vi "Process RS232 Messages.vi"(8 "error in (no error)":errorcluster, 10 "rt fifo":refnum<k33>, 11 "BMS RS232 STRING":string) -> (0 "error out":errorcluster, 2 "rt fifo out":refnum<k33>)   [LabVIEW 2015]
uses:
  1dstr.ctl
  <vilib>/RioEmbeddedCAN/RioEmbeddedCAN.llb/CANFrameControl.ctl
  Global Data.vi
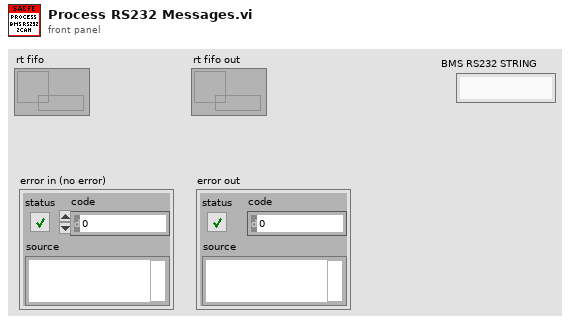
[diagram p1: front panel]
types:
  T1 = typedef "1dstr.ctl" = string[]
  T2 = typedef "CANFrameControl.ctl" = cluster{"identifier":u32, "extended?":bool, "type":u8, "payload":u8[]}
  T3 = typedef "BMS Telemetry.ctl" = cluster{"bBMSIgnition":bool, "bBMSChargerMains":bool, "bBMSFastCharge":bool, "bBMSChargerEnabled":bool, "eBMSCarState":enum16{"Off", "On, Not Charging", "Charging", "Charging Finished", "Charging Error"}, "eBMSChargingState":enum16{"Disconnected", "Pre-charging", "Main Charging", "Balancing", "Charging Finished OK", "Charging Error"}, "tBMSChargeStage":u16, "eBMSLastChargeError":enum16{"No Error", "No Cell Communication", "No Cell Communication - Non CAN Charger", "Maximum charging stage duration expired", "Cell Communication Lost during Charge", "Cannot set balancing voltage", "Cell temps too high", "No Comms so can't determine temp", "# of Cells Mismatch", "Cells Overvoltage", "Cell Protection Event occured."}, "NBMSNumCells":u8, "bBMSUnderVProtection":bool, "bBMSOverVProtection":bool, "bBMSOverTProtection":bool, "bBMSLeakageProtection":bool, "bBMSNoCellCommsError":bool, "bBMSLowVReduction":bool, "bBMSHighTReduction":bool, "VCellMin":dbl, "VCellMax":dbl, "VCellMean":dbl, "VTotal":dbl, "TCellMin":dbl, "TCellMax":dbl, "TCellMean":dbl, "VCells":cluster{"[51]":dbl, "[53]":dbl, "[54]":dbl, "[55]":dbl, "[56]":dbl, "[57]":dbl, "[58]":dbl, "[59]":dbl, "[60]":dbl, "[61]":dbl, "[62]":dbl, "[63]":dbl, "[64]":dbl, "[65]":dbl, "[66]":dbl, "[67]":dbl, "[34]":dbl, "[35]":dbl, "[36]":dbl, "[37]":dbl, "[38]":dbl, "[39]":dbl, "[40]":dbl, "[41]":dbl, "[42]":dbl, "[43]":dbl, "[44]":dbl, "[45]":dbl, "[46]":dbl, "[47]":dbl, "[48]":dbl, "[49]":dbl, "[50]":dbl, "[17]":dbl, "[18]":dbl, "[19]":dbl, "[20]":dbl, "[21]":dbl, "[22]":dbl, "[23]":dbl, "[24]":dbl, "[25]":dbl, "[26]":dbl, "[27]":dbl, "[28]":dbl, "[29]":dbl, "[30]":dbl, "[31]":dbl, "[32]":dbl, "[33]":dbl, "[0]":dbl, "[1]":dbl, "[2]":dbl, "[3]":dbl, "[4]":dbl, "[5]":dbl, "[6]":dbl, "[7]":dbl, "[8]":dbl, "[9]":dbl, "[10]":dbl, "[11]":dbl, "[12]":dbl, "[13]":dbl, "[14]":dbl, "[15]":dbl, "[16]":dbl, "[52] 2":dbl}, "TBMSCells":cluster{"[55]":dbl, "[56]":dbl, "[57]":dbl, "[58]":dbl, "[59]":dbl, "[60]":dbl, "[61]":dbl, "[62]":dbl, "[63]":dbl, "[64]":dbl, "[65]":dbl, "[66]":dbl, "[67]":dbl, "[68]":dbl, "[69]":dbl, "[70]":dbl, "[17]":dbl, "[38]":dbl, "[39]":dbl, "[40]":dbl, "[41]":dbl, "[42]":dbl, "[43]":dbl, "[44]":dbl, "[45]":dbl, "[46]":dbl, "[47]":dbl, "[48]":dbl, "[49]":dbl, "[50]":dbl, "[51]":dbl, "[52]":dbl, "[53]":dbl, "[54]":dbl, "[21]":dbl, "[22]":dbl, "[23]":dbl, "[24]":dbl, "[25]":dbl, "[26]":dbl, "[27]":dbl, "[28]":dbl, "[29]":dbl, "[30]":dbl, "[31]":dbl, "[32]":dbl, "[33]":dbl, "[34]":dbl, "[35]":dbl, "[36]":dbl, "[37]":dbl, "[0]":dbl, "[1]":dbl, "[2]":dbl, "[3]":dbl, "[4]":dbl, "[5]":dbl, "[6]":dbl, "[7]":dbl, "[8]":dbl, "[9]":dbl, "[10]":dbl, "[11]":dbl, "[12]":dbl, "[13]":dbl, "[14]":dbl, "[15]":dbl, "[16]":dbl}, "bChargerConnected":bool, "VChargerSetpoint":dbl, "IChargerSetpoint":dbl, "VChargerActual":dbl, "IChargerActual":dbl, "BCells":cluster{"[51]":dbl, "[52]":dbl, "[53]":dbl, "[54]":dbl, "[55]":dbl, "[56]":dbl, "[57]":dbl, "[58]":dbl, "[59]":dbl, "[60]":dbl, "[61]":dbl, "[62]":dbl, "[63]":dbl, "[64]":dbl, "[65]":dbl, "[66]":dbl, "[67]":dbl, "[34]":dbl, "[35]":dbl, "[36]":dbl, "[37]":dbl, "[38]":dbl, "[39]":dbl, "[40]":dbl, "[41]":dbl, "[42]":dbl, "[43]":dbl, "[44]":dbl, "[45]":dbl, "[46]":dbl, "[47]":dbl, "[48]":dbl, "[49]":dbl, "[50]":dbl, "[17]":dbl, "[18]":dbl, "[19]":dbl, "[20]":dbl, "[21]":dbl, "[22]":dbl, "[23]":dbl, "[24]":dbl, "[25]":dbl, "[26]":dbl, "[27]":dbl, "[28]":dbl, "[29]":dbl, "[30]":dbl, "[31]":dbl, "[32]":dbl, "[33]":dbl, "[0]":dbl, "[1]":dbl, "[2]":dbl, "[3]":dbl, "[4]":dbl, "[5]":dbl, "[6]":dbl, "[7]":dbl, "[8]":dbl, "[9]":dbl, "[10]":dbl, "[11]":dbl, "[12]":dbl, "[13]":dbl, "[14]":dbl, "[15]":dbl, "[16]":dbl}, "bNewVCellMinSample":bool, "Battery Temp":cluster{"[0]":dbl, "[1]":dbl, "[2]":dbl, "[3]":dbl, "[4]":dbl, "[5]":dbl, "[6]":dbl, "[7]":dbl, "[8]":dbl, "[9]":dbl, "[10]":dbl, "[11]":dbl, "[12]":dbl, "[13]":dbl, "[14]":dbl, "[15]":dbl, "[16]":dbl, "[0] 6":dbl, "[17]":dbl, "[18]":dbl, "[19]":dbl, "[20]":dbl, "[21]":dbl, "[22]":dbl, "[23]":dbl, "[24]":dbl, "[25]":dbl, "[26]":dbl, "[27]":dbl, "[28]":dbl, "[29]":dbl, "[30]":dbl, "[31]":dbl, "[32]":dbl, "[33]":dbl, "[17] 6":dbl, "[34]":dbl, "[35]":dbl, "[36]":dbl, "[37]":dbl, "[38]":dbl, "[39]":dbl, "[40]":dbl, "[41]":dbl, "[42]":dbl, "[43]":dbl, "[44]":dbl, "[45]":dbl, "[46]":dbl, "[47]":dbl, "[48]":dbl, "[49]":dbl, "[50]":dbl, "[34] 6":dbl, "[51]":dbl, "[52] 2":dbl, "[53]":dbl, "[54]":dbl, "[55]":dbl, "[56]":dbl, "[57]":dbl, "[58]":dbl, "[59]":dbl, "[60]":dbl, "[61]":dbl, "[62]":dbl, "[63]":dbl, "[64]":dbl, "[65]":dbl, "[66]":dbl, "[67]":dbl, "[51] 6":dbl, "[0] 2":dbl, "[1] 2":dbl, "[2] 2":dbl, "[3] 2":dbl, "[4] 2":dbl, "[5] 2":dbl, "[6] 2":dbl, "[7] 2":dbl, "[8] 2":dbl, "[9] 2":dbl, "[10] 2":dbl, "[11] 2":dbl, "[12] 2":dbl, "[13] 2":dbl, "[14] 2":dbl, "[15] 2":dbl, "[16] 2":dbl, "[0] 7":dbl, "[17] 2":dbl, "[18] 2":dbl, "[19] 2":dbl, "[20] 2":dbl, "[21] 2":dbl, "[22] 2":dbl, "[23] 2":dbl, "[24] 2":dbl, "[25] 2":dbl, "[26] 2":dbl, "[27] 2":dbl, "[28] 2":dbl, "[29] 2":dbl, "[30] 2":dbl, "[31] 2":dbl, "[32] 2":dbl, "[33] 2":dbl, "[17] 7":dbl, "[34] 2":dbl, "[35] 2":dbl, "[36] 2":dbl, "[37] 2":dbl, "[38] 2":dbl, "[39] 2":dbl, "[40] 2":dbl, "[41] 2":dbl, "[42] 2":dbl, "[43] 2":dbl, "[44] 2":dbl, "[45] 2":dbl, "[46] 2":dbl, "[47] 2":dbl, "[48] 2":dbl, "[49] 2":dbl, "[50] 2":dbl, "[34] 7":dbl, "[51] 2":dbl, "[52] 3":dbl, "[53] 2":dbl, "[54] 2":dbl, "[55] 2":dbl, "[56] 2":dbl, "[57] 2":dbl, "[58] 2":dbl, "[59] 2":dbl, "[60] 2":dbl, "[61] 2":dbl, "[62] 2":dbl, "[63] 2":dbl, "[64] 2":dbl, "[65] 2":dbl, "[66] 2":dbl, "[67] 2":dbl, "[51] 7":dbl, "[0] 3":dbl, "[1] 3":dbl, "[2] 3":dbl, "[3] 3":dbl, "[4] 3":dbl, "[5] 3":dbl, "[6] 3":dbl, "[7] 3":dbl, "[8] 3":dbl, "[9] 3":dbl, "[10] 3":dbl, "[11] 3":dbl, "[12] 3":dbl, "[13] 3":dbl, "[14] 3":dbl, "[15] 3":dbl, "[16] 3":dbl, "[0] 8":dbl, "[17] 3":dbl, "[18] 3":dbl, "[19] 3":dbl, "[20] 3":dbl, "[21] 3":dbl, "[22] 3":dbl, "[23] 3":dbl, "[24] 3":dbl, "[25] 3":dbl, "[26] 3":dbl, "[27] 3":dbl, "[28] 3":dbl, "[29] 3":dbl, "[30] 3":dbl, "[31] 3":dbl, "[32] 3":dbl, "[33] 3":dbl, "[17] 8":dbl, "[34] 3":dbl, "[35] 3":dbl, "[36] 3":dbl, "[37] 3":dbl, "[38] 3":dbl, "[39] 3":dbl, "[40] 3":dbl, "[41] 3":dbl, "[42] 3":dbl, "[43] 3":dbl, "[44] 3":dbl, "[45] 3":dbl, "[46] 3":dbl, "[47] 3":dbl, "[48] 3":dbl, "[49] 3":dbl, "[50] 3":dbl, "[34] 8":dbl, "[51] 3":dbl, "[52] 4":dbl, "[53] 3":dbl, "[54] 3":dbl, "[55] 3":dbl, "[56] 3":dbl, "[57] 3":dbl, "[58] 3":dbl, "[59] 3":dbl, "[60] 3":dbl, "[61] 3":dbl, "[62] 3":dbl, "[63] 3":dbl, "[64] 3":dbl, "[65] 3":dbl, "[66] 3":dbl, "[67] 3":dbl, "[51] 8":dbl, "[0] 4":dbl, "[1] 4":dbl, "[2] 4":dbl, "[3] 4":dbl, "[4] 4":dbl, "[5] 4":dbl, "[6] 4":dbl, "[7] 4":dbl, "[8] 4":dbl, "[9] 4":dbl, "[10] 4":dbl, "[11] 4":dbl, "[12] 4":dbl, "[13] 4":dbl, "[14] 4":dbl, "[15] 4":dbl, "[16] 4":dbl, "[0] 9":dbl, "[17] 4":dbl, "[18] 4":dbl, "[19] 4":dbl, "[20] 4":dbl, "[21] 4":dbl, "[22] 4":dbl, "[23] 4":dbl, "[24] 4":dbl, "[25] 4":dbl, "[26] 4":dbl, "[27] 4":dbl, "[28] 4":dbl, "[29] 4":dbl, "[30] 4":dbl, "[31] 4":dbl, "[32] 4":dbl, "[33] 4":dbl, "[17] 9":dbl, "[34] 4":dbl, "[35] 4":dbl, "[36] 4":dbl, "[37] 4":dbl, "[38] 4":dbl, "[39] 4":dbl, "[40] 4":dbl, "[41] 4":dbl, "[42] 4":dbl, "[43] 4":dbl, "[44] 4":dbl, "[45] 4":dbl, "[46] 4":dbl, "[47] 4":dbl, "[48] 4":dbl, "[49] 4":dbl, "[50] 4":dbl, "[34] 9":dbl, "[51] 4":dbl, "[52] 5":dbl, "[53] 4":dbl, "[54] 4":dbl, "[55] 4":dbl, "[56] 4":dbl, "[57] 4":dbl, "[58] 4":dbl, "[59] 4":dbl, "[60] 4":dbl, "[61] 4":dbl, "[62] 4":dbl, "[63] 4":dbl, "[64] 4":dbl, "[65] 4":dbl, "[66] 4":dbl, "[67] 4":dbl, "[51] 9":dbl}, "TBMSMax":dbl, "TBMSMin":dbl, "TBMSMean":dbl}
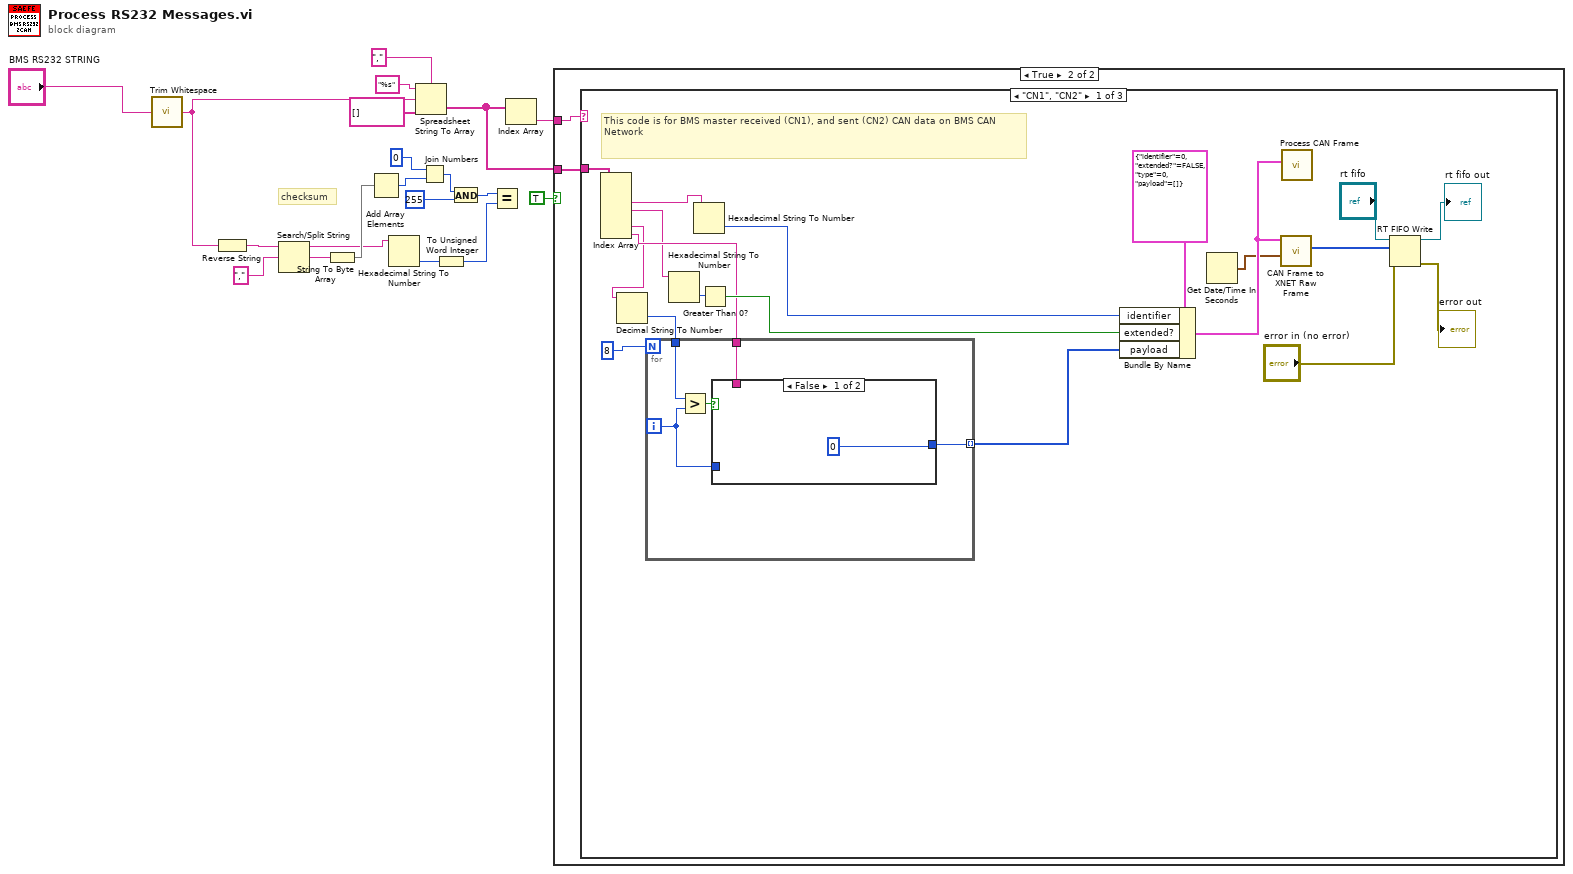
[diagram p0: block diagram]
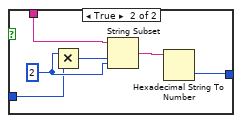
[diagram p3: hidden frame]
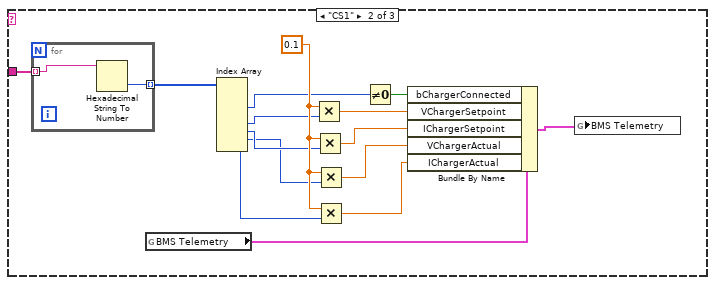
[diagram p4: hidden frame]
diagram:
  # "checksum"
  n1 = call <vilib>:"Trim Whitespace.vi"("string"="BMS RS232 STRING") -> ("trimmed string"=w12:string)  [unwired: 1 in]
  n2 = Reverse String(1:w12) -> (0:w11:string)
  n3 = Search/Split String(string=w11, search string/char (-)=",") -> (substring before match=w8:string, match + rest of string=w10:string)  [unwired: 1 in, 1 out]
  n4 = String To Byte Array(string=w10) -> (unsigned byte array=w9:u8[])
  n5 = Add Array Elements(numeric array=w9) -> (sum=w6:u8)
  n6 = Hexadecimal String To Number(string=w8) -> (number=w4:u32)  [unwired: 2 in, 1 out]
  n7 = Spreadsheet String To Array(delimiter (Tab)=",", format string="%s", spreadsheet string=w12, array type (2D Dbl)=T1 [] ("String")) -> (array=w14:string[])
  n8 = Join Numbers(hi=u8 0, lo=w6) -> ((hi.lo)=w7:u16)
  n9 = To Unsigned Word Integer(number=w4) -> (unsigned 16bit integer=w3:u16)
  n10 = And(x=w7, y=u16 255) -> (x .and. y?=w19:u16)
  n11 = Equal?(x=w19, y=w3) -> ()  [unwired: 1 out]
  n12 = Index Array(array=w14) -> (element=w15:string)  [unwired: 1 in]
  n13 = case shown="True" TRUE {
    tunnel: w15 -> [_ w22]
    tunnel: w14 -> [_ w21]
    frame False {
    }
    frame True {
      n14 = case shown="\"CN1\", \"CN2\"" w22 {
        tunnel: w21 -> [w41 w68 _]
        frame "CN1", "CN2" {
          # "This code is for BMS master received (CN1), and sent (CN2) CAN data on BMS CAN Network"
          n15 = Index Array(array=w41) -> (element #2=w32:string, element #3=w33:string, element #5=w34:string, element #6=w35:string)  [unwired: 6 in, 2 out]
          n16 = Decimal String To Number(string=w34) -> (number=w30:i32)  [unwired: 2 in, 1 out]
          n17 = for {
            N: 8 -> [_]
            tunnel: w35 -> [w46]
            tunnel: [w45] -> w36 mode=indexing
            tunnel: w30 -> [w44]
            i -> [w43]
            n18 = Greater?(x=w44, y=w43) -> (0:w42:bool)
            n19 = case shown="False" w42 {
              tunnel: w46 -> [_ w53]
              tunnel: [u8 0 w49] -> w45
              tunnel: w43 -> [_ w48]
              frame False {
              }
              frame True {
                w51 = 2
                n20 = Multiply(x=w51, y=w48) -> (x*y=w52:i32)
                n21 = String Subset(string=w53, offset (0)=w52, length (rest)=w51) -> (substring=w50:string)
                n22 = Hexadecimal String To Number(string=w50) -> (number=w49:u32)  [unwired: 2 in, 1 out]
              }
            }
          }
          n23 = Hexadecimal String To Number(string=w33) -> (number=w40:u32)  [unwired: 2 in, 1 out]
          n24 = Hexadecimal String To Number(string=w32) -> (number=w38:u32)  [unwired: 2 in, 1 out]
          n25 = Greater Than 0?(x=w40) -> (x > 0?=w37:bool)
          n26 = Bundle By Name(cluster=T2 {"identifier"=0, "extended?"=FALSE, "type"=0, "payload"=[]} ("CAN frame"), "identifier"=w38, "extended?"=w37, "payload"=w36) -> (w29:T2)
          n27 = Get Date/Time In Seconds() -> (seconds since 1Jan1904=w23:timestamp)
          n28 = call "CAN Frame to XNET Raw Frame.vi"("timestamp"=w23, "CAN frame"=w29) -> ("Raw Frame"=w28:u8[])  [unwired: 8 in, 1 out]
          n29 = call "Process CAN Frame.vi"("CAN frame"=w29) -> ()  [unwired: 11 in]
          n30 = RT FIFO Write(0:"rt fifo", 1:w28, 3:"error in (no error)") -> (8:→"rt fifo out":refnum<k33>, 11:→"error out":errorcluster)  [unwired: 2 in, 2 out]
        }
        frame "CS1" {
          w63 = 0.1 ("x")
          n31 = for {
            tunnel: w68 -> [w70] mode=indexing
            tunnel: [w69] -> w67 mode=indexing
            n32 = Hexadecimal String To Number(string=w70) -> (number=w69:u32)  [unwired: 2 in, 1 out]
          }
          n33 = global read "Global Data.vi" "BMS Telemetry"() -> (w66:T3)
          n34 = Index Array(array=w67) -> (element #2=w58:u32, element #4=w57:u32, element #5=w56:u32, element #6=w55:u32, element #7=w54:u32)  [unwired: 7 in, 2 out]
          n35 = Multiply(x=w63, y=w57) -> (x*y=w64:dbl)
          n36 = Multiply(x=w63, y=w56) -> (x*y=w62:dbl)
          n37 = Multiply(x=w63, y=w55) -> (x*y=w61:dbl)
          n38 = Multiply(x=w63, y=w54) -> (x*y=w60:dbl)
          n39 = Not Equal To 0?(x=w58) -> (x != 0?=w65:bool)
          n40 = Bundle By Name(cluster=w66, "bChargerConnected"=w65, "VChargerSetpoint"=w64, "IChargerSetpoint"=w62, "VChargerActual"=w61, "IChargerActual"=w60) -> (w59:T3)
          n41 = global write "Global Data.vi" "BMS Telemetry"(w59) -> ()
        }
        frame Default {
        }
      }
    }
  }
